vi "Write OVP_Enable.vi"(8 "error in":errorcluster, 10 "OVP_Enable":bool, 11 "69X_79X in":refnum<class "69X_79X.lvclass">) -> (0 "error out":errorcluster, 3 "69X_79X out":refnum<class "69X_79X.lvclass">)   [LabVIEW 2019, in "69X_79X.lvlib" / "69X_79X.lvclass"]
uses:
  Library/69X_79X.lvclass
  builds/Instruments/PowerSupply.lvlibp/Library/PowerSupply.lvclass
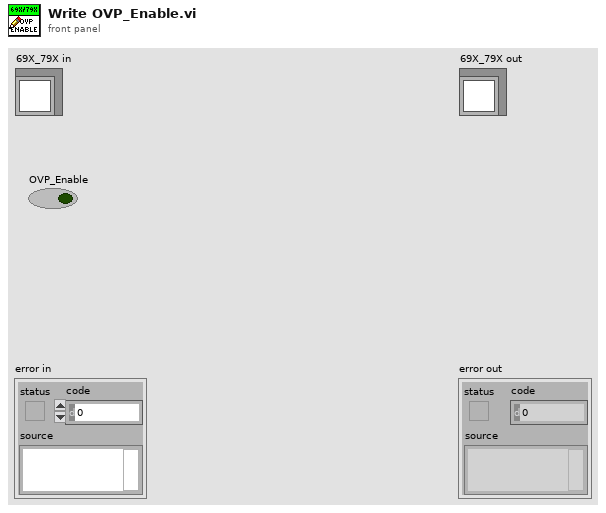
[diagram p1: front panel]
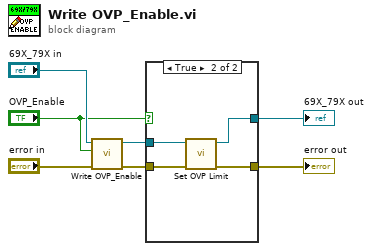
[diagram p0: block diagram]
diagram:
  n1 = call-parent "Write OVP_Enable.vi"("error in"="error in", "OVP_Enable"="OVP_Enable", "PowerSupply in"="69X_79X in") -> ("error out"=w3:errorcluster, "PowerSupply out"=w4:refnum<class "69X_79X.lvclass">)  [unwired: 7 in]
  n2 = case shown="True" "OVP_Enable" {
    tunnel: w4 -> [w9 w12]
    tunnel: w3 -> [w8 w13]
    tunnel: [w9 w11] -> w2
    tunnel: [w8 w10] -> w1
    frame False {
    }
    frame True {
      n3 = call "Set OVP Limit.vi"("error in"=w13, "69X_79X in"=w12) -> ("error out"=w10:errorcluster, "69X_79X out"=w11:refnum<class "69X_79X.lvclass">)  [unwired: 8 in]
    }
  }
  "error out" <- w1
  "69X_79X out" <- w2
